vi "Get Telemetry Config.vi"(8 "error in (no error)":errorcluster, 11 "Node Config in":refnum<class "Node Config.lvclass">) -> (0 "error out":errorcluster, 2 "Telemtry Config":T1, 3 "Node Config out":refnum<class "Node Config.lvclass">)   [LabVIEW 2020, in "VectoConfig.lvlib" / "Node Config.lvclass"]
uses:
  Node Config.lvclass
  VectoConfig/Telemetry Config.ctl
  VectoConfig/Telemetry Routing.ctl
  VectoConfig/Endpoint.ctl
  Node Config.lvclass/Node Config.ctl
  VectoConfig/VectoConfig.lvlib
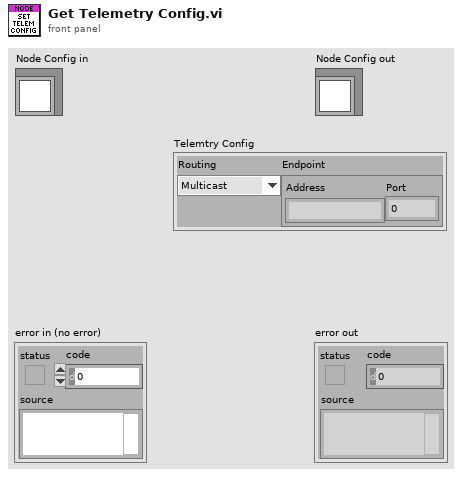
[diagram p1: front panel]
types:
  T1 = typedef "VectoConfig.lvlib/Telemetry Config.ctl" = cluster{"Routing":T2, "Endpoint":T3}
  T2 = typedef "VectoConfig.lvlib/Telemetry Routing.ctl" = enum16{"Multicast", "Unicast"}
  T3 = typedef "VectoConfig.lvlib/Endpoint.ctl" = cluster{"Address":string, "Port":u16}
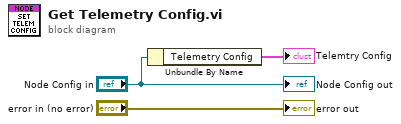
[diagram p0: block diagram]
diagram:
  n1 = Unbundle By Name("Node Config in") -> ("Telemetry Config"=→"Telemtry Config":T1)
  "error out" <- "error in (no error)"
  "Node Config out" <- "Node Config in"
